vi "New MemberAttendance.vi"(6 "AttendanceData":string[][](array[string]), 7 "CurWeek(0)":i32, 8 "error in (no error)":errorcluster, 9 "Department(\"\")":string, 10 "Name(\"\")":string, 11 "MemberAttendance in":refnum<class "MemberAttendance.lvclass">) -> (0 "error out":errorcluster, 3 "MemberAttendance out":refnum<class "MemberAttendance.lvclass">)   [LabVIEW 2015, in "Admin_Actor.lvlib" / "MemberAttendance.lvclass"]
uses:
  MemberAttendance.lvclass
  MemberAttendance.lvclass/MemberAttendance.ctl
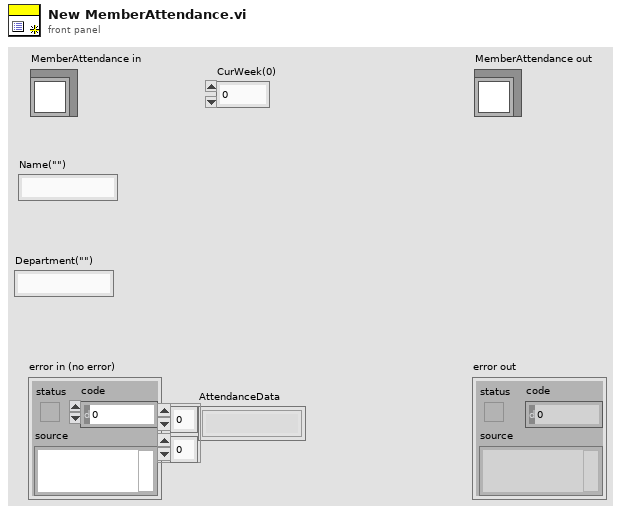
[diagram p1: front panel]
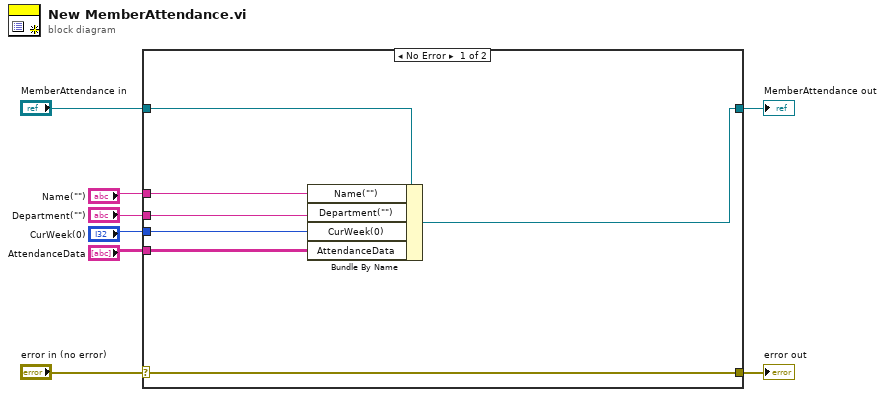
[diagram p0: block diagram]
diagram:
  n1 = case shown="No Error" "error in (no error)" {
    selector: "error in (no error)" -> [w15 w17]
    tunnel: [w15 w17] -> w7
    tunnel: [w13 w16] -> w5
    tunnel: "MemberAttendance in" -> [w14 w16]
    tunnel: "Name(\"\")" -> [w12 _]
    tunnel: "Department(\"\")" -> [w11 _]
    tunnel: "CurWeek(0)" -> [w10 _]
    tunnel: "AttendanceData" -> [w9 _]
    frame No Error {
      n2 = Bundle By Name(cluster=w14, "Name(\"\")"=w12, "Department(\"\")"=w11, "CurWeek(0)"=w10, "AttendanceData"=w9) -> (w13:refnum<class "MemberAttendance.lvclass">)
    }
    frame Error {
    }
  }
  "error out" <- w7
  "MemberAttendance out" <- w5
